vi "Parse Certificate Info.vi"(7 "message body":string, 11 "error in (no error)":errorcluster) -> (4 "certificates":T1(array[cluster]), 15 "error out":errorcluster)   [LabVIEW 2016]
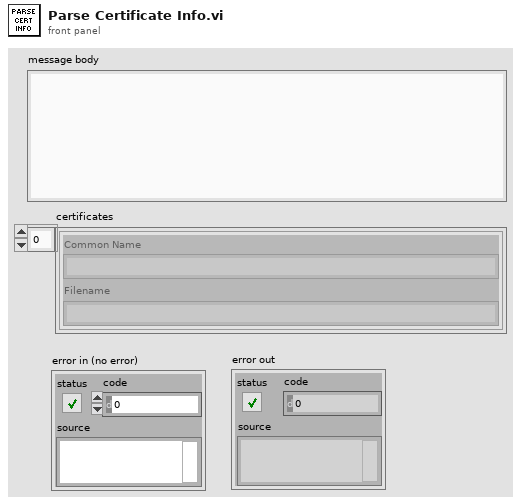
[diagram p1: front panel]
types:
  T1 = cluster{"Common Name":string, "Filename":string}[]
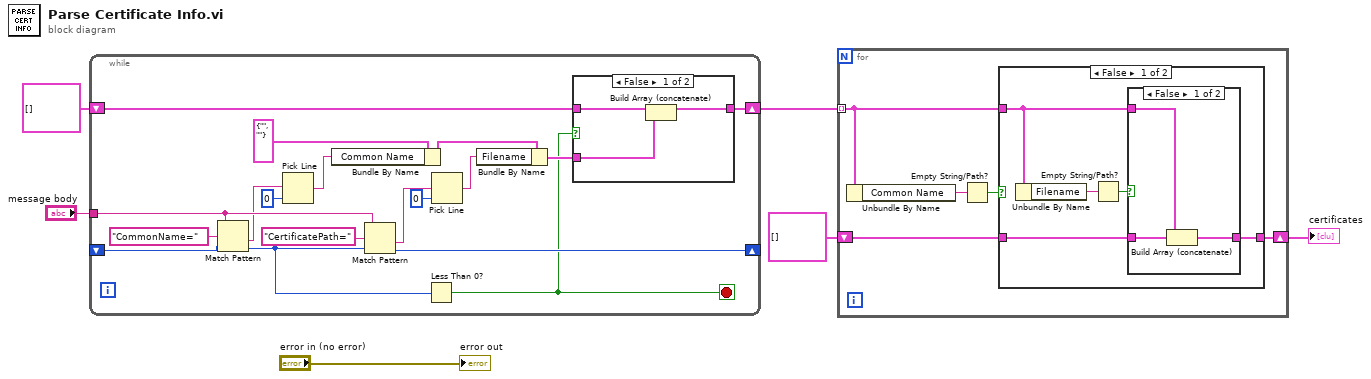
[diagram p0: block diagram]
diagram:
  n1 = while {
    tunnel: "message body" -> [w22]
    shift-right: [w9] -> _
    shift-left: _ -> [w19]
    shift-right: [w11] -> w4
    shift-left: T1 [] -> [w10]
    stop <- w7 stop-if-true
    n2 = Match Pattern(string=w22, regular expression="CommonName=", offset (0)=w19) -> (after substring=w21:string, offset past match=w8:i32)  [unwired: 2 out]
    n3 = Pick Line(multi-line string=w21, line index=0) -> (output string=w18:string)  [unwired: 1 in]
    n4 = Bundle By Name(cluster=cluster{"Common Name":string, "Filename":string} {"Common Name"="", "Filename"=""} ("Cluster"), "Common Name"=w18) -> (w16:cluster{"Common Name":string, "Filename":string})
    n5 = Match Pattern(string=w22, regular expression="CertificatePath=", offset (0)=w8) -> (after substring=w20:string, offset past match=w9:i32)  [unwired: 2 out]
    n6 = Less Than 0?(x=w8) -> (x < 0?=w7:bool)
    n7 = Pick Line(multi-line string=w20, line index=0) -> (output string=w17:string)  [unwired: 1 in]
    n8 = Bundle By Name(cluster=w16, "Filename"=w17) -> (w12:cluster{"Common Name":string, "Filename":string})
    n9 = case shown="False" w7 {
      tunnel: w12 -> [w27 _]
      tunnel: [w26 w28] -> w11
      tunnel: w10 -> [w25 w28]
      frame False {
        n10 = Build Array (concatenate)(w25, w27) -> (w26:T1)
      }
      frame True {
      }
    }
  }
  n11 = for {
    tunnel: w4 -> [w31] mode=indexing
    shift-right: [w30] -> w2
    shift-left: T1 [] -> [w29]
    n12 = Unbundle By Name(w31) -> ("Common Name"=w33:string)
    n13 = Empty String/Path?(string/path=w33) -> (empty?=w32:bool)
    n14 = case shown="False" w32 {
      tunnel: w31 -> [w36 _]
      tunnel: [w35 w43] -> w30
      tunnel: w29 -> [w34 w43]
      frame False {
        n15 = Unbundle By Name(w36) -> ("Filename"=w38:string)
        n16 = Empty String/Path?(string/path=w38) -> (empty?=w37:bool)
        n17 = case shown="False" w37 {
          tunnel: w36 -> [w41 _]
          tunnel: [w40 w42] -> w35
          tunnel: w34 -> [w39 w42]
          frame False {
            n18 = Build Array (concatenate)(w41, w39) -> (w40:T1)
          }
          frame True {
          }
        }
      }
      frame True {
      }
    }
  }
  "certificates" <- w2
  "error out" <- "error in (no error)"
